vi "Return client handle.vi"(8 "error in (no error)":errorcluster, 9 "headers":T1[](array[typedef]), 10 "Client Handle":T2, 11 "REST Client in":refnum<class "REST Client_JKI.lvclass">) -> (0 "error out":errorcluster, 3 "REST Client out":refnum<class "REST Client_JKI.lvclass">)   [LabVIEW 2018, in "REST Client.lvlib" / "REST Client_JKI.lvclass"]
uses:
  REST Client_JKI.lvclass
  <vilib>/httpClient/ClientHandle.ctl
  REST Client/HTTP Header.ctl
  REST Client_JKI.lvclass/REST Client_JKI.ctl
  <vilib>/httpClient/LabVIEWHTTPClient.lvlib
  REST Client/REST Client.lvclass
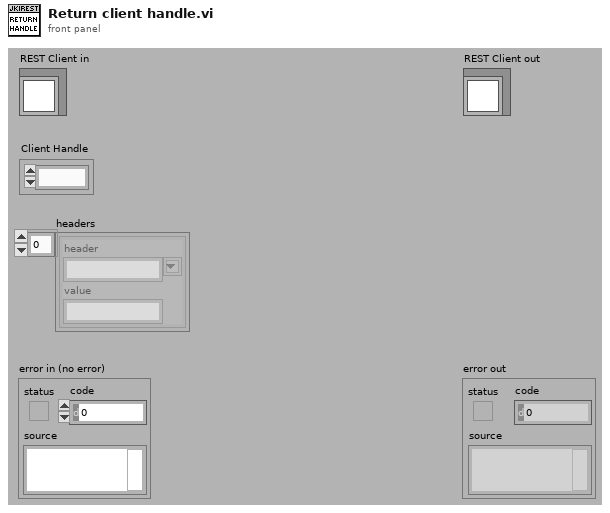
[diagram p1: front panel]
types:
  T1 = typedef "REST Client.lvlib/REST Client.lvclass/HTTP Header.ctl" = cluster{"header":string, "value":string}
  T2 = typedef "LabVIEWHTTPClient.lvlib/ClientHandle.ctl" = refnum<k1>
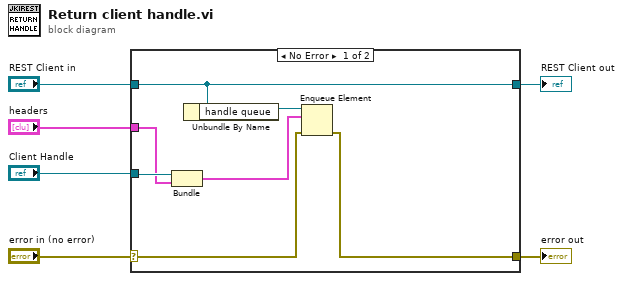
[diagram p0: block diagram]
diagram:
  n1 = case shown="No Error" "error in (no error)" {
    selector: "error in (no error)" -> [w9 w14]
    tunnel: [w8 w14] -> w5
    tunnel: [w11 w15] -> w3
    tunnel: "REST Client in" -> [w11 w15]
    tunnel: "Client Handle" -> [w13 _]
    tunnel: "headers" -> [w12 _]
    frame No Error {
      n2 = Bundle("Client Handle"=w13, "headers"=w12) -> (w7:cluster{"Client Handle":T2, "headers":T1[]})  [unwired: 1 in]
      n3 = Unbundle By Name(w11) -> ("handle queue"=w10:refnum<queue>)
      n4 = Enqueue Element(queue=w10, element=w7, error in (no error)=w9) -> (error out=w8:errorcluster)  [unwired: 1 in, 2 out]
    }
    frame Error {
    }
  }
  "error out" <- w5
  "REST Client out" <- w3
